vi "Reset Timer.vi"(9 "Branched Timer Index":T2, 11 "NXT":T1={"Hardware"="NXT", "Flattened String"=""}) -> (3 "NXT":T1={"Hardware"="NXT", "Flattened String"=""})   [LabVIEW 2010, in "timerExts.lvlib"]
uses:
  timerExts.lvlib
  Branched Timer.ctl
  <vilib>/NXT/Subs/LVHSConnector.ctl
  CLIB/CRef/Interface/CRef Numeric.llb/U32 CReference.ctl
  CLIB/CRef/CRef.lvlib
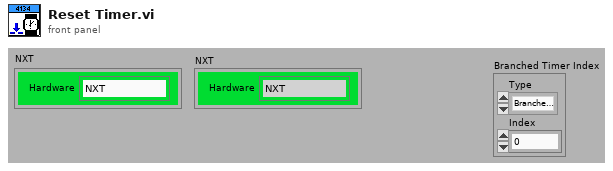
[diagram p1: front panel]
types:
  T1 = typedef "LVHSConnector.ctl" = cluster{"Hardware":string, "Flattened String":string}
  T2 = typedef "timerExts.lvlib/Branched Timer.ctl" = cluster{"Type":enum8{"Branched Timer", "NXT Timer"}, "Index":u16}
  T3 = typedef "CRef.lvlib/U32 CReference.ctl" = cluster{"Generic CRef Address":u16, "Type":enum8{"Null", "Boolean", "U8", "I8", "U16", "I16", "U32", "I32", "U64", "I64", "Single", "Double", "Extended", "CSG", "CDB", "CXT", "Invalid Def", "U8(Def)", "I8(Def)", "U16(Def)", "I16(Def)", "U32(Def)"}}
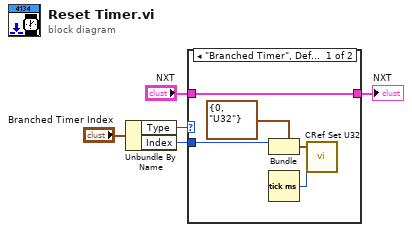
[diagram p0: block diagram]
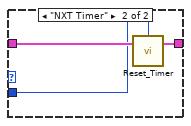
[diagram p2: hidden frame]
diagram:
  n1 = Unbundle By Name("Branched Timer Index") -> ("Type"=w4:enum8{"Branched Timer", "NXT Timer"}, "Index"=w3:u16)
  n2 = case shown="\"Branched Timer\", Default" w4 {
    tunnel: w3 -> [w7 w11]
    tunnel: "NXT" -> [w10 w13]
    tunnel: [w10 w12] -> w1
    frame "Branched Timer", Default {
      n3 = Bundle(cluster=T3 {"Generic CRef Address"=0, "Type"=enum."U32"} ("U32 CReference"), "Generic CRef Address"=w7) -> (w8:T3)  [unwired: 1 in]
      n4 = Tick Count (ms)() -> (millisecond timer value=w6:u32)
      n5 = call "CRef Set U32.vi"("Value"=w6, "U32 CReference"=w8) -> ()  [unwired: 3 in, 1 out]
    }
    frame "NXT Timer" {
      n6 = call <vilib>:"Reset_Timer.vi"("NXT"=w13, "Timer (Timer 1)"=w11) -> ("NXT"=w12:T1)  [unwired: 2 in]
    }
  }
  "NXT" <- w1
